vi "TEST_004.vi"() -> ()   [LabVIEW 2014]
doc: "This example is for the LEGO MINDSTORMS NXT. The program utilizes proportional control to keep an robotic arm at a constant distance above a surface using only a light sensor at the distal end of the arm to measure position."
uses:
  <vilib>/NXT/Block Support/NXT_OutputPort.ctl
  <vilib>/NXT/NXTIO Xnodes/NXTIONodeSubVIs/NXTMoveMotors.vi
  <vilib>/NXT/Dual Mode Library/Waits/Wait_Num.vi
  <vilib>/NXT/NXTIO Xnodes/NXTIONodeSubVIs/LEGOResetMotors.vi
  <vilib>/NXT/NXTIO Xnodes/NXTIONodeSubVIs/LEGOMotorStatus.vi
  <vilib>/NXT/Dual Mode Library/Waits/Wait_Num(msec).vi
  <vilib>/NXT/NXTIO Xnodes/NXTIONodeSubVIs/NXTStopMotors.vi
  <vilib>/NXT/Subs/LVHSConnector.ctl
  <vilib>/NXT/NXTIO Xnodes/AddressXNode/NXTIOAddress.xnode
  <vilib>/NXT/NXTIO Xnodes/NXTIOXNode/NXTIO.xnode
  <vilib>/NXT/LegoClasses/BrickReference/BrickReference.lvclass
  DLLFIRST.dll
panel:
  in  "숫자형 5":dbl
  out "숫자형 4":dbl
  out "숫자형 3":dbl
  out "숫자형 2":dbl
  out "숫자형":dbl
  out "场":dbl
  out "시작":dbl
  in  "MODE":dbl
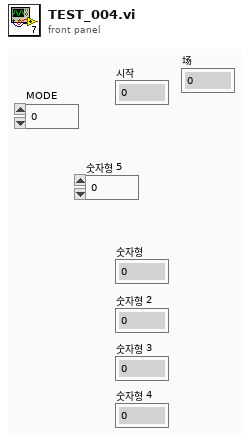
[diagram p1: front panel]
types:
  T1 = typedef "NXT_OutputPort.ctl" = u8
  T2 = cluster{"Output Port":T1, "Output Port 2":T1, "Output Port 3":T1}
  T3 = typedef "LVHSConnector.ctl" = refnum<class "BrickReference.lvclass">
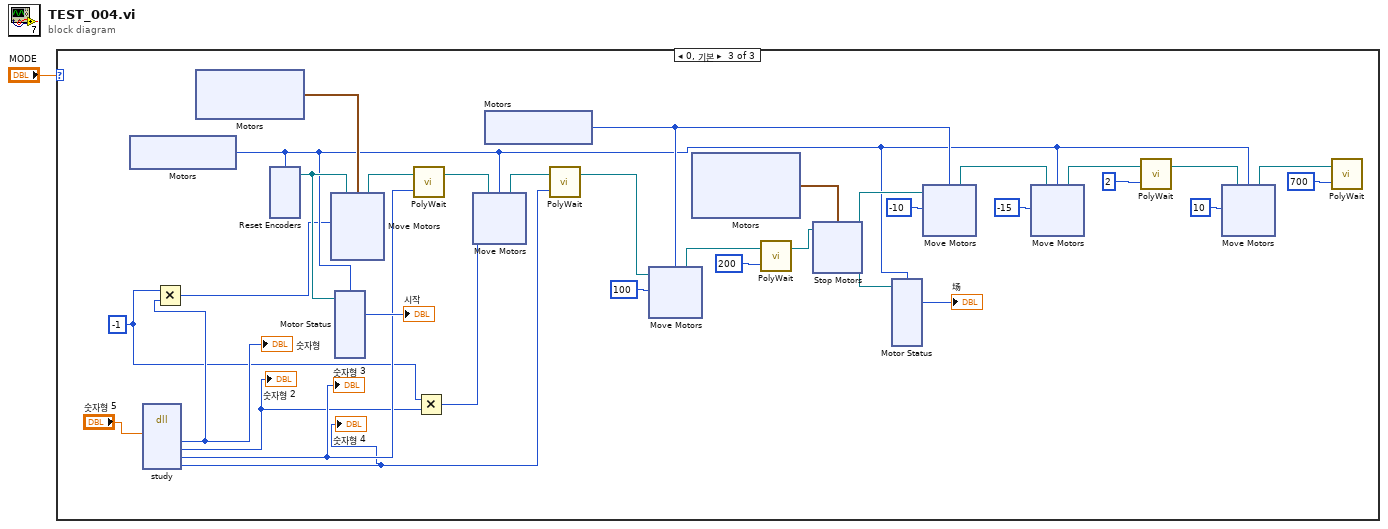
[diagram p0: block diagram]
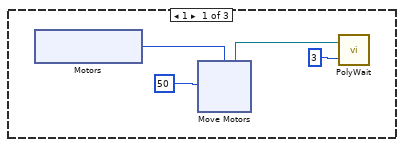
[diagram p2: hidden frame]
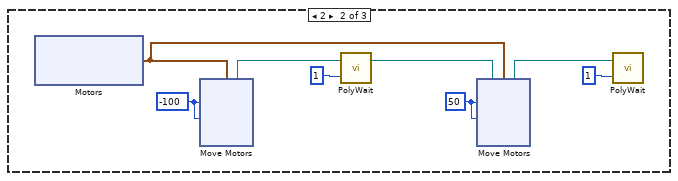
[diagram p3: hidden frame]
diagram:
  n1 = case shown="0, 기본" "MODE" {
    frame 1 {
      n2 = xnode "Motors"() -> ("Motor"=w5:T1)
      n3 = xnode "Move Motors"("Power/Speed 1"=50, "Motors"=w5) -> ("NXT/EV3"=w2:T3)  [unwired: 1 in]
      n4 = call-poly <vilib>:"PolyWait.vi"("Time (1 sec)"=3, "NXT/EV3"=w2) -> ()  [unwired: 2 in, 1 out]
    }
    frame 2 {
      w19 = 50
      w16 = -100
      n5 = xnode "Motors"() -> ("Motor"=w17:cluster{"Port":T1, "Port":T1})
      n6 = xnode "Move Motors"("Power/Speed 2"=w16, "Power/Speed 1"=w16, "Motors"=w17) -> ("NXT/EV3"=w14:T3)  [unwired: 1 in]
      n7 = call-poly <vilib>:"PolyWait.vi"("Time (1 sec)"=1, "NXT/EV3"=w14) -> ("NXT/EV3"=w18:T3)  [unwired: 2 in]
      n8 = xnode "Move Motors"("Power/Speed 2"=w19, "Power/Speed 1"=w19, "Motors"=w17, "NXT/EV3"=w18) -> ("NXT/EV3"=w21:T3)
      n9 = call-poly <vilib>:"PolyWait.vi"("Time (1 sec)"=1, "NXT/EV3"=w21) -> ()  [unwired: 2 in, 1 out]
    }
    frame 0, Default {
      w41 = -1
      n10 = xnode "Motors"() -> ("Motor"=w48:T1)
      n11 = dll-call lib="PTH2:abs CUsers\t과학고Desktop2015 R&EDLLFIRST.dll" fn="study"("state"="숫자형 5") -> ("w1"=w43:i32, "w2"=w42:i32, "t2"=w46:i32, "t3"=w45:i32)  [unwired: 9 in, 2 out]
      "숫자형" <- w43
      "숫자형 2" <- w42
      "숫자형 3" <- w46
      "숫자형 4" <- w45
      n12 = Multiply(x=w41, y=w43) -> (x*y=w44:i32)
      n13 = xnode "Motors"() -> ("Motor"=w71:cluster{"Port":T1, "Port":T1})
      n14 = xnode "Reset Encoders"("Motors"=w48) -> ("NXT/EV3"=w58:T3)  [unwired: 1 in]
      n15 = xnode "Move Motors"("Power/Speed 2"=w44, "Power/Speed 1"=w44, "Motors"=w71, "NXT/EV3"=w58) -> ("NXT/EV3"=w69:T3)
      n16 = xnode "Motor Status"("Motors"=w48, "NXT/EV3"=w58) -> ("Position 1"=→"시작":i32)  [unwired: 2 out]
      n17 = call-poly <vilib>:"PolyWait.vi"("Time (100 msec)"=w46, "NXT/EV3"=w69) -> ("NXT/EV3"=w68:T3)  [unwired: 2 in]
      n18 = Multiply(x=w41, y=w42) -> (x*y=w40:i32)
      n19 = xnode "Move Motors"("Power/Speed 1"=w40, "Motors"=w48, "NXT/EV3"=w68) -> ("NXT/EV3"=w67:T3)
      n20 = xnode "Motors"() -> ("Motor"=w63:T1)
      n21 = call-poly <vilib>:"PolyWait.vi"("Time (100 msec)"=w45, "NXT/EV3"=w67) -> ("NXT/EV3"=w66:T3)  [unwired: 2 in]
      n22 = xnode "Move Motors"("Power/Speed 1"=100, "Motors"=w63, "NXT/EV3"=w66) -> ("NXT/EV3"=w65:T3)
      n23 = xnode "Motors"() -> ("Motor"=w59:cluster{"Port":T1, "Port":T1, "Port":T1})
      n24 = call-poly <vilib>:"PolyWait.vi"("Time (100 msec)"=200, "NXT/EV3"=w65) -> ("NXT/EV3"=w61:T3)  [unwired: 2 in]
      n25 = xnode "Stop Motors"("Motors"=w59, "NXT/EV3"=w61) -> ("NXT/EV3"=w56:T3)
      n26 = xnode "Motor Status"("Motors"=w48, "NXT/EV3"=w56) -> ("Position 1"=→"场":i32)  [unwired: 2 out]
      n27 = xnode "Move Motors"("Power/Speed 1"=-10, "Motors"=w63, "NXT/EV3"=w56) -> ("NXT/EV3"=w53:T3)
      n28 = xnode "Move Motors"("Power/Speed 1"=-15, "Motors"=w48, "NXT/EV3"=w53) -> ("NXT/EV3"=w52:T3)
      n29 = call-poly <vilib>:"PolyWait.vi"("Time (1 sec)"=2, "NXT/EV3"=w52) -> ("NXT/EV3"=w50:T3)  [unwired: 2 in]
      n30 = xnode "Move Motors"("Power/Speed 1"=10, "Motors"=w48, "NXT/EV3"=w50) -> ("NXT/EV3"=w49:T3)
      n31 = call-poly <vilib>:"PolyWait.vi"("Time (100 msec)"=700, "NXT/EV3"=w49) -> ()  [unwired: 2 in, 1 out]
    }
  }
